vi "扫码枪.vi"() -> ()   [LabVIEW 2018]
panel:
  in  "条码":string
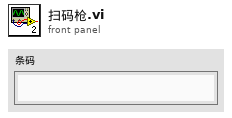
[diagram p1: front panel]
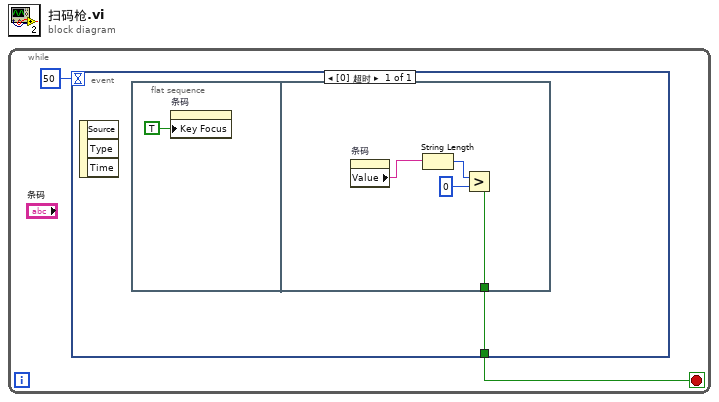
[diagram p0: block diagram]
diagram:
  n1 = while {
    stop <- w1 stop-if-true
    n2 = event shown="[0] 超时" {
      selector: _ -> [_]
      dyn-events: _ -> [_]
      timeout: 50 -> [_]
      tunnel: [w3] -> w1
      event Timeout {
        n3 = event-data() -> ()  [unwired: 1 in, 3 out]
        n4 = flat-sequence {
          tunnel: [w5] -> w3
          frame #0 {
            n5 = property on="条码" class="Str"("Key Focus"=TRUE) -> ()  [unwired: 2 in, 2 out]
          }
          frame #1 {
            n6 = property on="条码" class="Str"() -> ("Value"=w8:string)  [unwired: 2 in, 2 out]
            n7 = String Length(string=w8) -> (length=w7:i32)
            n8 = Greater?(x=w7, y=0) -> (0:w5:bool)
          }
        }
      }
    }
  }
